vi "Ref AVI Video-Get refs.vi"(8 "error in (no error)":errorcluster, 11 "Timelapse count":u32) -> (0 "error out":errorcluster, 1 "Ref Y Length":u32, 2 "AVI mode":T5, 3 "Ref X Length":u32, 4 "Green PMT is ON":bool, 5 "Red AVI":T1, 6 "Green AVI":T1, 7 "Red PMT is ON":bool)   [LabVIEW 2020]
uses:
  Typedefs/AVI implementation enum.ctl
  Typedefs/AVI Refs cluster.ctl
  <vilib>/vision/Avi.llb/IMAQ AVI2 Refnum.ctl
  <vilib>/vision/Image Controls.llb/IMAQ Image.ctl
  <vilib>/vision/Avi1.llb/AviRefnum.ctl
panel:
  # "SUBROUTINE VI"
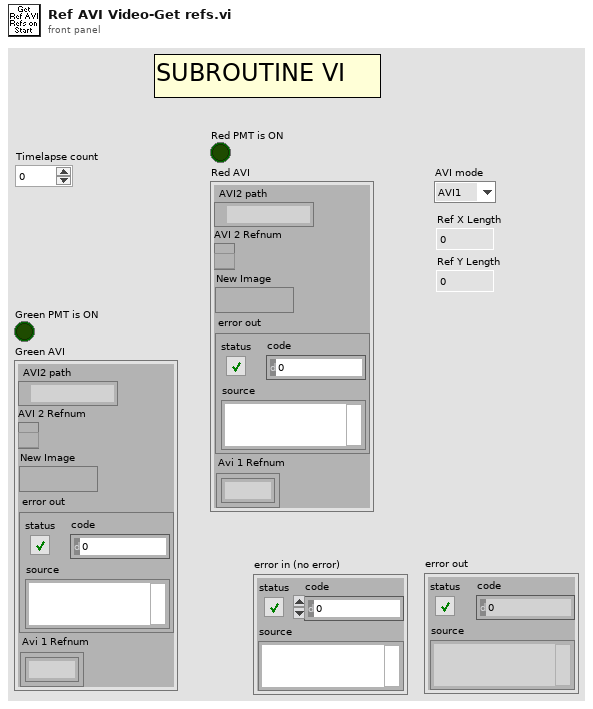
[diagram p1: front panel]
types:
  T1 = typedef "AVI Refs cluster.ctl" = cluster{"AVI2 path":path, "AVI 2 Refnum":T2, "New Image":T3, "error out":errorcluster, "Avi 1 Refnum":T4}
  T2 = typedef "IMAQ AVI2 Refnum.ctl" = refnum<k20>
  T3 = typedef "IMAQ Image.ctl" = refnum<image>
  T4 = typedef "AviRefnum.ctl" = refnum<k1>
  T5 = typedef "AVI implementation enum.ctl" = enum16{"AVI1", "AVI2"}
  T6 = cluster{"AVI mode":T5, "Red Ref AVI":T1, bool, "Green Ref AVI":T1, bool, u32, u32}
  T7 = typedef "Ref DAQ Param.ctl" = cluster{"Full Frame Size":u16, "Ref Field of View":sgl, "Ref Zoom":i8, "Ref_dwellTime":sgl, "Ref X-pixels-per-line(Npxr)":i16, "Ref Y-lines-per-image(Npyr)":i16, "Ref Z-lines-per-image":i16, "Ignore Z lines":i16, "Ref Scan Cycles":i32, "Ref threshold XY":u16, "Ref threshold Z":u16, "Ref average XY":u16, "Ref Average  Z":u16, "Proportional_scale":fxp<+,16,2>, "Integral_scale":fxp<+/-,16,12>, "Proportional_scale Z":fxp<+,16,2>, "Integral_scale Z":fxp<+/-,16,12>, "Diff_threshold":fxp<+,16,2>, "Diff_threshold _z":fxp<+,16,2>, "Sliding Average":bool, "Ref count reset enabled":bool}
  T8 = typedef "AOL_Globals.ctl" = cluster{"Imaging Protocol":T9, "Number of POI":u16, "Number of Miniscans":u16, "Number of Trials":u16, "Number of Cycles ":u64, "# Averaged Frames":u16, "Laser power (%)":u8, "Pockels (V)":dbl, "Acquisition Length (sec)":dbl, "Fill time (us)":dbl, "POI Dwell time (us)":dbl, "Miniscan Dwell time per pixel (us)":dbl, "PMT 1":dbl, "PMT 2":dbl, "Back Apperture (mA)":dbl, "Frame Size":T10, "Center Frequency":dbl, "Field of View (norm)":dbl, "DwellTime (us)":dbl, "Wavelength (nm)":dbl, "Zoom":dbl, "AOL Z":dbl, "AOL Mode":T11, "GridXY":dbl, "GridZ":dbl, "TriggerPeriod (sec)":dbl, "Number of Pixels in Miniscan":u16, "Experiment folder path":path, "X centre":dbl, "Y centre":dbl, "Angle (degrees)":dbl, "Plane Mode":T12, "Threshold":u16[], "Regenerate Chirps":bool, "Rectangle ROI length (pixels)":u16, "Rectangle ROI height (pixels)":u16, "AOD fill":u16, "StartupDelay":i32, "Samples Wait after Trigger":u16, "Slip Cycle":u32, "Add Cycle":bool, "Functional Mode":T13, "Z Start":dbl, "Z Stop":dbl, "# Planes":i32, "Total Pixels":i32, "Variable Miniscan Pixels":u16[], "Use Variable Length":bool, "Use Variable Resolution":bool, "Laser power (%) at Z Start":u8, "Laser power (%) at Z Stop":u8, "Ref Z Step":i8, "Ref Dwell Time (us)":dbl, "Field of View (um)":dbl}
  T9 = typedef "Imaging Protocols enum.ctl" = enum16{"AOL Z-Stack", "Motor Z Stack", "Functional Acquisition", "Single Plane Acquisition", "Volume Acquisition", "Live Imaging", "Live Plane Imaging", "Live Volume Imaging"}
  T10 = typedef "Frame Size.ctl" = u16
  T11 = typedef "AOL modes.ctl" = enum16{"Raster", "Structural", "Pointing", "Mini Scan", "Alignment"}
  T12 = typedef "Plane Mode.ctl" = u16
  T13 = typedef "Functional Mode.ctl" = enum16{"Point", "Line", "Patch", "Plane", "Volume"}
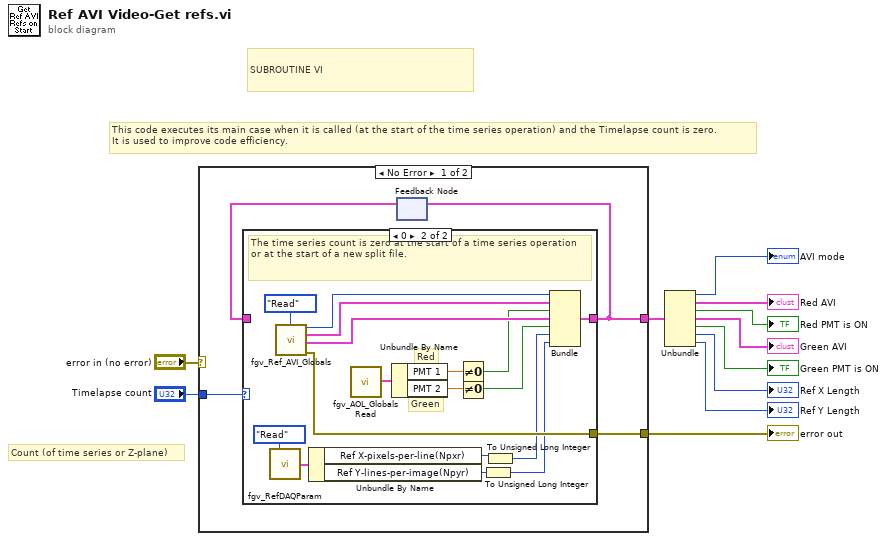
[diagram p0: block diagram]
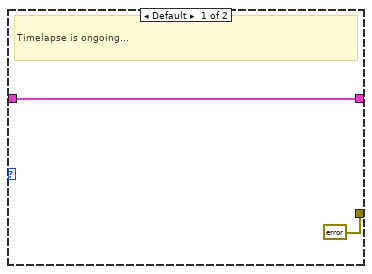
[diagram p2: hidden frame]
diagram:
  # "Count (of time series or Z-plane)"
  # "SUBROUTINE VI"
  # "This code executes its main case when it is called (at the start of the time series operation) and the Timelapse count is zero.\nIt is used to improve code efficiency."
  n1 = case shown="No Error" "error in (no error)" {
    selector: "error in (no error)" -> [_ w35]
    tunnel: [w15 _] -> w6
    tunnel: [w13 w35] -> w4
    tunnel: "Timelapse count" -> [w12 _]
    frame No Error {
      n2 = feedback #1() -> (w14:T6)  [unwired: 1 in]
      n3 = case shown="0" w12 {
        tunnel: [w17 w30] -> w15
        tunnel: w14 -> [w17 _]
        tunnel: [errorcluster {"status"=FALSE, "code"=0, "source"=""} ("error out") w29] -> w13
        frame Default {
          # "Timelapse is ongoing..."
        }
        frame 0 {
          # "Green"
          # "Red"
          # "The time series count is zero at the start of a time series operation or at the start of a new split file."
          n4 = call "fgv_RefDAQParam.vi"("Function"=enum16{"Initialize", "Write", "Read"}."Read" ("Status")) -> ("RefDAQParam"=w28:T7)  [unwired: 9 in, 1 out]
          n5 = call "fgv_Ref_AVI_Globals.vi"("Function"=enum16{"Intialize", "Write", "Read", "Clear"}."Read") -> ("AVI mode"=w33:T5, "Red Ref AVI"=w32:T1, "Green Ref AVI"=w31:T1, "error out"=w29:errorcluster)  [unwired: 11 in]
          n6 = Unbundle By Name(w28) -> ("Ref X-pixels-per-line(Npxr)"=w27:i16, "Ref Y-lines-per-image(Npyr)"=w26:i16)
          n7 = call "fgv_AOL_Globals Read.vi"() -> ("AOL_Globals"=w20:T8)  [unwired: 9 in, 2 out]
          n8 = Unbundle By Name(w20) -> ("PMT 1"=w19:dbl, "PMT 2"=w18:dbl)
          n9 = Not Equal To 0?(x=w19) -> (x != 0?=w22:bool)
          n10 = Not Equal To 0?(x=w18) -> (x != 0?=w21:bool)
          n11 = To Unsigned Long Integer(number=w26) -> (unsigned 32bit integer=w24:u32)
          n12 = To Unsigned Long Integer(number=w27) -> (unsigned 32bit integer=w25:u32)
          n13 = Bundle("AVI mode"=w33, "Red Ref AVI"=w32, w22, "Green Ref AVI"=w31, w21, w25, w24) -> (w30:T6)  [unwired: 1 in]
        }
      }
      n14 = feedback-in #1(w15) -> ()
    }
    frame Error {
    }
  }
  "error out" <- w4
  n15 = Unbundle(w6) -> ("AVI mode"=→"AVI mode":T5, "Red Ref AVI"=→"Red AVI":T1, →"Red PMT is ON":bool, "Green Ref AVI"=→"Green AVI":T1, →"Green PMT is ON":bool, →"Ref X Length":u32, →"Ref Y Length":u32)
